vi "from string.vi"(8 "error in":errorcluster, 9 "data":string, 10 "version":string, 11 "configuration in":refnum<class "Bus Configuration.lvclass">) -> (0 "error out":errorcluster, 3 "configuration out":refnum<class "Bus Configuration.lvclass">)   [LabVIEW 2014, in "Bus Configuration.lvclass"]
doc: "Provides an interface for loading a module configuration from a file or other serialized data source. It is recommended that all children of this class store data in two sets--data required for its own initialization, and any data required for parent initialization--and that each implementation uses the <b>Call Parent Method</b> primitive to de-serialize parent information."
uses:
  Bus Configuration.lvclass
  SPI Configuration.ctl
  Bus Configuration.lvclass/Bus Configuration.ctl
  <vilib>/NI/Configuration Framework/serializable configuration/NISE_CEF_serializable configuration.lvclass
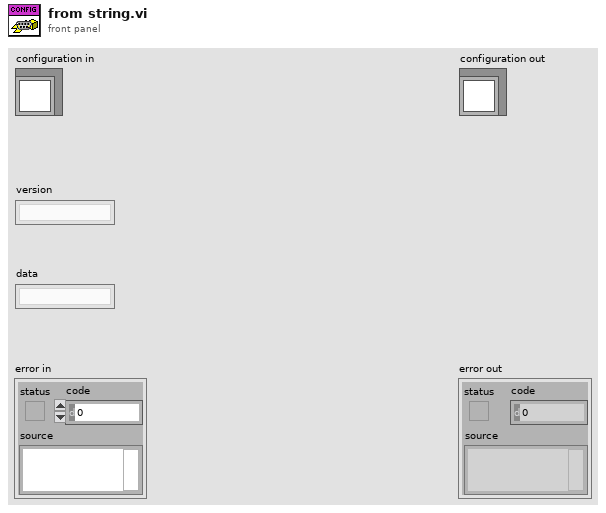
[diagram p1: front panel]
types:
  T1 = typedef "Bus Configuration.lvclass/SPI Configuration.ctl" = cluster{"SCLK":string, "MOSI":string, "MISO":string}
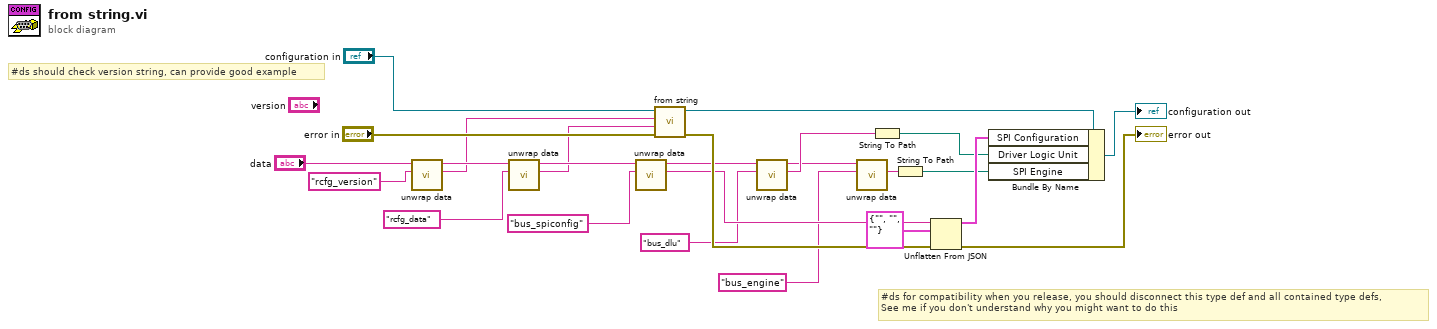
[diagram p0: block diagram]
diagram:
  # "#ds for compatibility when you release, you should disconnect this type def and all contained type defs,\nSee me if you don't understand why you might want to do this"
  # "#ds should check version string, can provide good example"
  n1 = call <vilib>:"unwrap data.vi"("identifier"="rcfg_version" ("additional identifier"), "data to unwrap"="data") -> ("unwrapped data"=w16:string, "remaining string"=w22:string)  [unwired: 8 in]
  n2 = call <vilib>:"unwrap data.vi"("identifier"="rcfg_data" ("additional identifier"), "data to unwrap"=w22) -> ("unwrapped data"=w15:string, "remaining string"=w20:string)  [unwired: 8 in]
  n3 = call <vilib>:"unwrap data.vi"("identifier"="bus_spiconfig" ("additional identifier"), "data to unwrap"=w20) -> ("unwrapped data"=w9:string, "remaining string"=w8:string)  [unwired: 8 in]
  n4 = call-parent "from string.vi"("error in"="error in", "data"=w15, "version"=w16, "configuration in"="configuration in") -> ("error out"=w12:errorcluster, "configuration out"=w14:refnum<class "Bus Configuration.lvclass">)  [unwired: 6 in]
  n5 = call <vilib>:"unwrap data.vi"("identifier"="bus_dlu", "data to unwrap"=w8) -> ("unwrapped data"=w7:string, "remaining string"=w2:string)  [unwired: 8 in]
  n6 = call <vilib>:"unwrap data.vi"("identifier"="bus_engine", "data to unwrap"=w2) -> ("unwrapped data"=w3:string)  [unwired: 8 in, 1 out]
  n7 = String To Path(string=w7) -> (path=w6:path)
  n8 = String To Path(string=w3) -> (path=w1:path)
  n9 = Unflatten From JSON(JSON string=w9, type and defaults=T1 {"SCLK"="", "MOSI"="", "MISO"=""} ("SPI Configuration"), error in (no error)=w12) -> (value=w13:T1, error out=→"error out":errorcluster)  [unwired: 4 in]
  n10 = Bundle By Name(cluster=w14, "SPI Configuration"=w13, "Driver Logic Unit"=w6, "SPI Engine"=w1) -> (→"configuration out":refnum<class "Bus Configuration.lvclass">)
